vi "get channels.vi"(11 "Modbus Slave configuration in":refnum<class "Modbus Slave configuration.lvclass">) -> (2 "channels":refnum<class "TBM channel.lvclass">[](array[class]), 3 "Modbus Slave configuration out":refnum<class "Modbus Slave configuration.lvclass">)   [LabVIEW 2013, in "Modbus Slave configuration.lvclass"]
doc: "Platypus Framework 1.0.1.65\nNI Systems Engineering - National Instruments"
uses:
  Modbus Slave configuration.lvclass
  <vilib>/NI/Tag Bus Module Framework/channel/TBM channel.lvclass
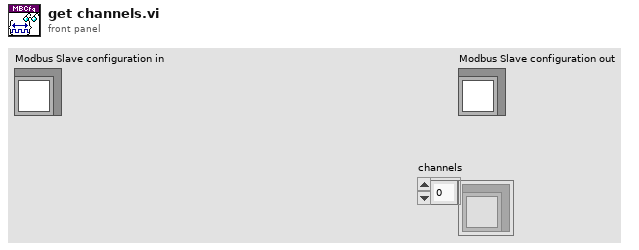
[diagram p1: front panel]
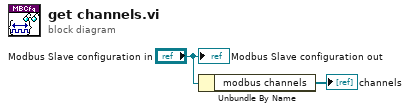
[diagram p0: block diagram]
diagram:
  n1 = Unbundle By Name("Modbus Slave configuration in") -> ("modbus channels"=→"channels":refnum<class "Modbus Module Channel.lvclass">[])
  "Modbus Slave configuration out" <- "Modbus Slave configuration in"
